vi "LHF.DB.Mongo.Collection.FindOneById.vi"(6 "Extract _id (T)":bool=TRUE, 7 "type":variant, 8 "error in (no error)":errorcluster, 9 "_id":string, 10 "Collection":string, 11 "LHF.DB.Mongo in":refnum<class "LHF.DB.Mongo.lvclass">) -> (0 "error out":errorcluster, 1 "_id":string, 2 "Document":variant, 3 "LHF.DB.Mongo out":refnum<class "LHF.DB.Mongo.lvclass">)   [LabVIEW 2013, in "LHF.DB.Mongo.lvclass"]
uses:
  LHF.DB.Mongo.lvclass
  C:/Users/Ricardo/Desktop/Projetos/LabVIEW-MongoDB/src/Driver/MongoDB.Bson.dll
  Driver/MongoDB.Bson.dll
  C:/Users/Ricardo/Desktop/Projetos/LabVIEW-MongoDB/src/Driver/MongoDB.Driver.dll
  Driver/MongoDB.Driver.dll
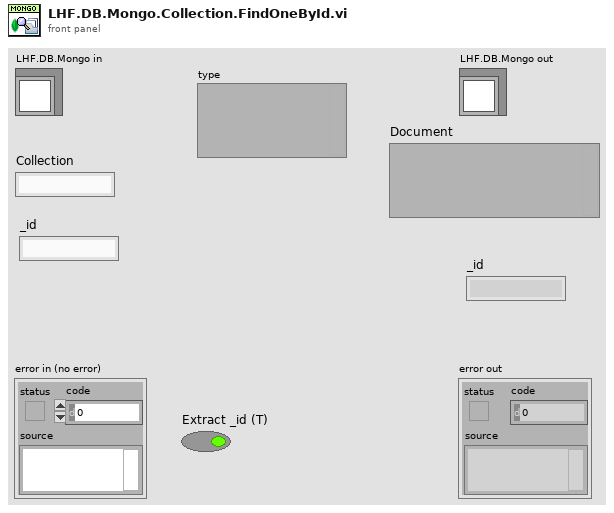
[diagram p1: front panel]
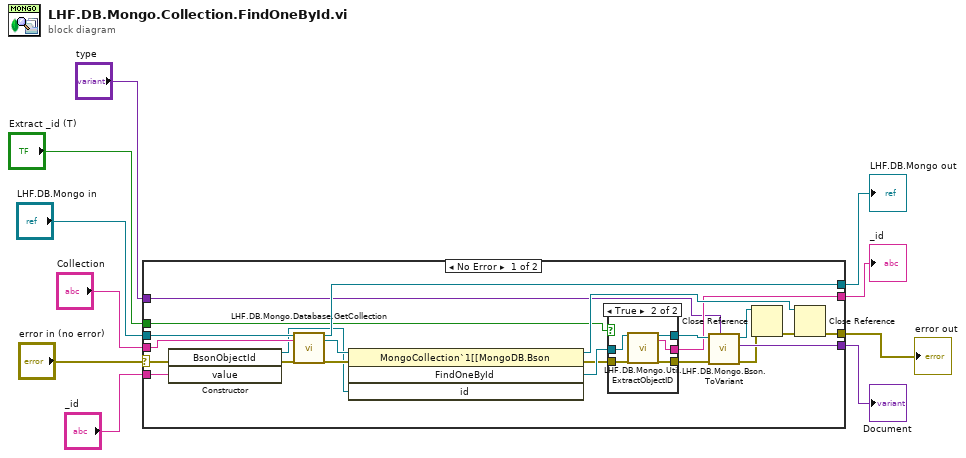
[diagram p0: block diagram]
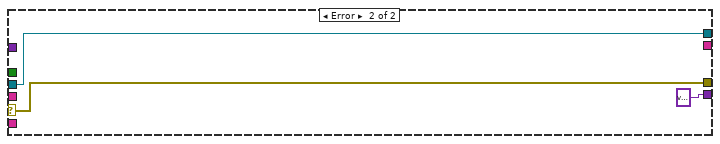
[diagram p3: hidden frame]
diagram:
  n1 = case shown="No Error" "error in (no error)" {
    selector: "error in (no error)" -> [w18 w42]
    tunnel: [w28 w42] -> w1
    tunnel: [w31 w41] -> w8
    tunnel: "LHF.DB.Mongo in" -> [w30 w41]
    tunnel: "Collection" -> [w32 _]
    tunnel: [w21 _] -> w6
    tunnel: "_id" -> [w20 _]
    tunnel: "Extract _id (T)" -> [w16 _]
    tunnel: "type" -> [w13 _]
    tunnel: [w12 variant ("data")] -> w2
    frame No Error {
      n2 = constructor class="BsonObjectId"(error in=w18, "value"=w20) -> (reference out=w19:refnum<k24>, error out=w17:errorcluster)  [unwired: 2 in, 2 out]
      n3 = call "LHF.DB.Mongo.Database.GetCollection.vi"("LHF.DB.Mongo in"=w30, "collectionName"=w32, "error in (no error)"=w17) -> ("LHF.DB.Mongo in"=w31:refnum<class "LHF.DB.Mongo.lvclass">, "MongoCollection"=w27:refnum<k24>, "error out"=w26:errorcluster)  [unwired: 14 in]
      n4 = invoke class="MongoCollection`1[[MongoDB.Bson" method="FindOneById"(reference=w27, error in=w26, "id"=w19) -> (reference out=w29:refnum<k24>, error out=w15:errorcluster, "FindOneById"=w23:refnum<k24>)  [unwired: 1 in, 1 out]
      n5 = case shown="True" w16 {
        tunnel: [w34 w39] -> w25
        tunnel: [w33 w38] -> w14
        tunnel: w23 -> [w34 w37]
        tunnel: [_ w36] -> w21
        tunnel: w15 -> [w33 w35]
        frame False {
        }
        frame True {
          n6 = call "LHF.DB.Mongo.Util.ExtractObjectID.vi"("BsonDocument Refnum in"=w37, "error in (no error)"=w35) -> ("BsonDocument Refnum out"=w39:refnum<k24>, "_id"=w36:string, "error out"=w38:errorcluster)  [unwired: 15 in]
        }
      }
      n7 = call "LHF.DB.Mongo.Bson.ToVariant.vi"("type"=w13, "error in (no error)"=w14, "BsonValue"=w25) -> ("error out"=w11:errorcluster, "data"=w12:variant, "BsonValue 2"=w24:refnum<k24>)  [unwired: 6 in]
      n8 = Close Reference(reference=w24, error in (no error)=w11) -> (error out=w22:errorcluster)
      n9 = Close Reference(reference=w29, error in (no error)=w22) -> (error out=w28:errorcluster)
    }
    frame Error {
    }
  }
  "error out" <- w1
  "LHF.DB.Mongo out" <- w8
  "Document" <- w2
  "_id" <- w6
